vi "禹山电导率_设置用户校准参数.vi"(8 "error in (no error)":errorcluster caption="错误输入（无错误）", 10 "用户校准参数":cluster{"K":sgl, "B":sgl}, 11 "MB session in":refnum<class "MB_Master.lvclass">) -> (0 "error out":errorcluster caption="错误输出", 3 "MB session out":refnum<class "MB_Master.lvclass">)   [LabVIEW 2016, in "斯坦道多参数.lvlib"]
uses:
  <vilib>/Plasmionique/MB Master/MB Master.lvlib
  <vilib>/Plasmionique/MB Master/MB_Master/MB_Master.lvclass
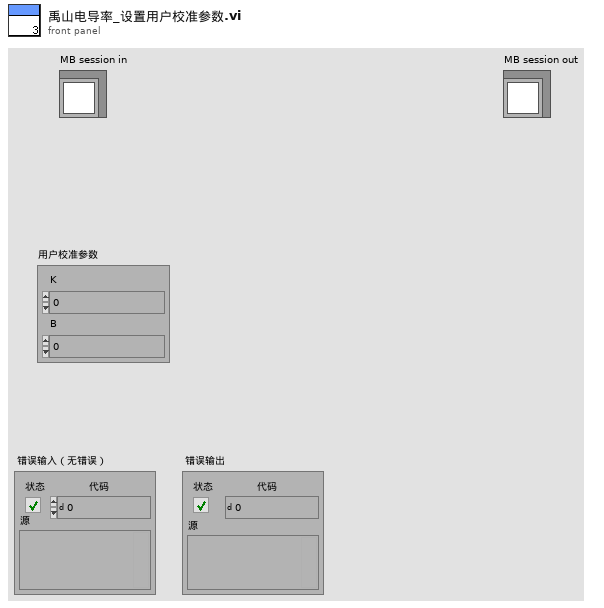
[diagram p1: front panel]
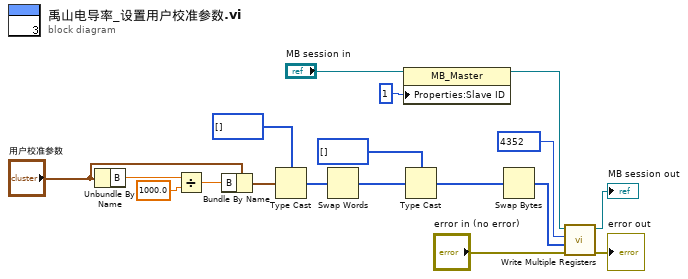
[diagram p0: block diagram]
diagram:
  n1 = Unbundle By Name("用户校准参数") -> ("B"=w3:sgl)
  n2 = Divide(x=w3, y=sgl 1000.0) -> (x/y=w2:sgl)
  n3 = Bundle By Name(cluster="用户校准参数", "B"=w2) -> (w4:cluster{"K":sgl, "B":sgl})
  n4 = Type Cast(type=u32[] [] ("数组 2"), x=w4) -> (*(type *) &x=w8:u32[])
  n5 = Swap Words(1:w8) -> (0:w12:u32[])
  n6 = property class="MB_Master"(reference="MB session in", "Properties:Slave ID"=u8 1 ("Slave ID")) -> (reference out=w15:refnum<class "MB_Master.lvclass">)  [unwired: 1 in, 1 out]
  n7 = Type Cast(type=u16[] [] ("数组 2"), x=w12) -> (*(type *) &x=w11:u16[])
  n8 = Swap Bytes(anything=w11) -> (byte swapped=w9:u16[])
  n9 = call <vilib>:"Write Multiple Registers.vi"("error in (no error)"="error in (no error)", "values"=w9, "starting address"=u16 4352, "MB session in"=w15) -> ("error out"=→"error out":errorcluster, "MB session out"=→"MB session out":refnum<class "MB_Master.lvclass">)  [unwired: 6 in]
